vi "Extracted algo.vi"(0 "Image In":T2, 2 "Match Options (Shape Detection 1)":T1={"Rotation"=FALSE, "Scale"=FALSE, "Occlusion"=TRUE, "Range Settings"=[{"Match Constraints"=2, "Min"=0.0, "Max"=50.0}]} {"Range Settings"."Match Constraints" items=["Rotation Angle (degrees)", "Scale Factor (%)", "Occlusion (%)"]}, 3 "Range (Threshold 1)":cluster{"Lower value":sgl, "Upper value":sgl}={"Lower value"=0.0, "Upper value"=195.0}, 7 "error in":errorcluster) -> (20 "Image Out":T2, 21 "Circles (Shape Detection 1)":T3(array[cluster]) {"Position"."Y" format="%.2f"; "Position"."X" format="%.2f"}, 22 "Circles Calibrated (Shape Detection 1)":T3(array[cluster]) {"Position"."Y" format="%.2f"; "Position"."X" format="%.2f"}, 23 "Number of Matches (Shape Detection 1)":i32, 27 "error out":errorcluster)   [LabVIEW 2015]
doc: "Creates, edits, and runs vision algorithms using NI Vision Assistant.\n\nWhen you place this Express VI on the block diagram, NI Vision Assistant launches. Create an algorithm using the Vision Assistant processing functions. After you create an algorithm, you can select the controls and indicators that you want to be able to programmatically set in LabVIEW. Double-click the Vision Assistant Express VI to edit the algorithm."
uses:
  <vilib>/vision/Image Controls.llb/IMAQ Image.ctl
  algo1.vi
  <vilib>/vision/NI_Vision_Development_Module.lvlib
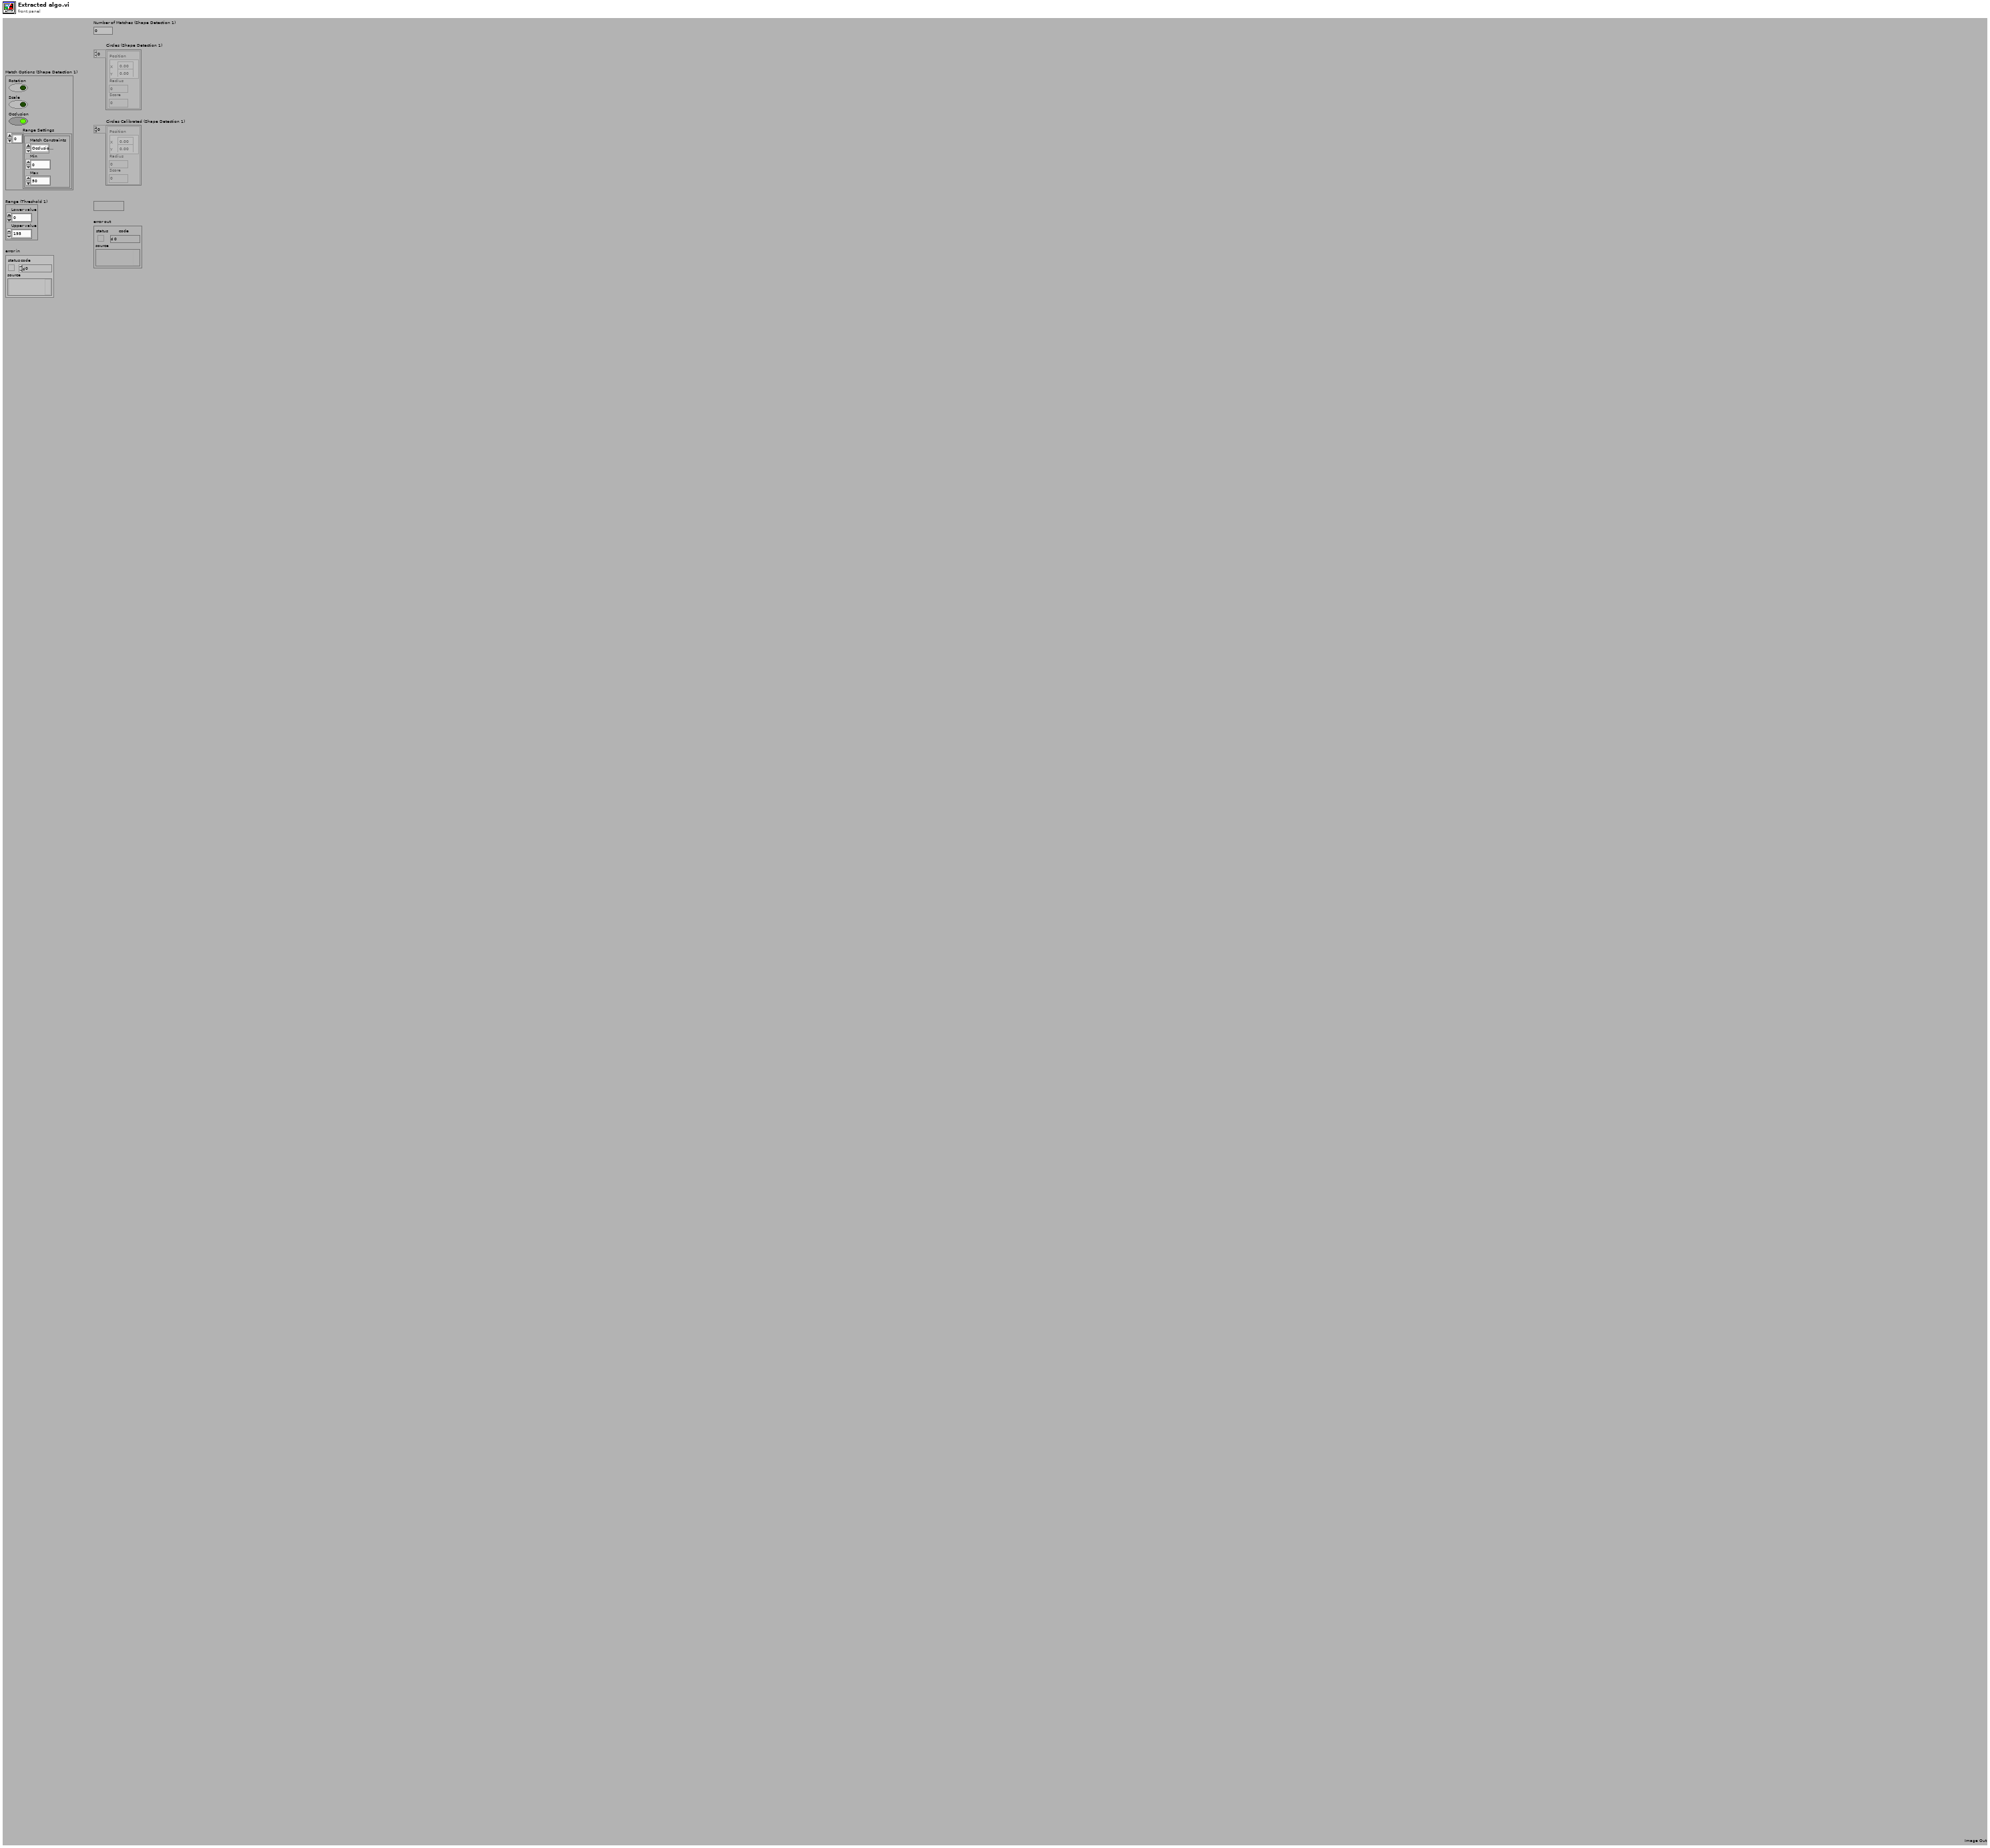
[diagram p1: front panel]
types:
  T1 = cluster{"Rotation":bool, "Scale":bool, "Occlusion":bool, "Range Settings":cluster{"Match Constraints":u32, "Min":dbl, "Max":dbl}[]}
  T2 = typedef "IMAQ Image.ctl" = refnum<image>
  T3 = cluster{"Position":cluster{"X":sgl, "Y":sgl}, "Radius":dbl, "Score":dbl}[]
  T4 = cluster{"Extraction Mode":u32, "Edge Threshold":i32, "Edge Filter Size":u32, "Min Length":i32, "Row Search Step Size":i32, "Col Search Step Size":i32, "Max Endpoint Gap":i32, "Closed":bool, "Subpixel":bool}
  T5 = cluster{"Global Rectangle":i32[], "Contours":cluster{"ID":enum32{"External", "Internal"}, "Type":u32, "Coordinates":i32[]}[]}
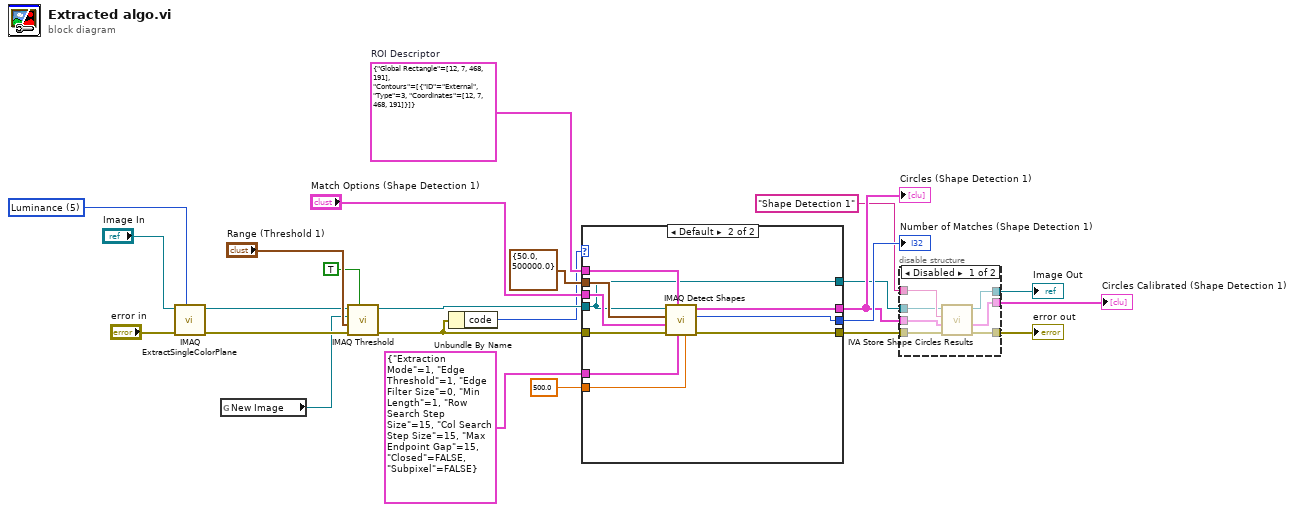
[diagram p0: block diagram]
diagram:
  w13 = T5 {"Global Rectangle"=[12, 7, 468, 191], "Contours"=[{"ID"=enum."External", "Type"=3, "Coordinates"=[12, 7, 468, 191]}]}  # ROI Descriptor
  w24 = 5 items=["Red", "Green", "Blue", "Hue", "Saturation", "Luminance", "Value", "Intensity"] ("Color Plane")
  n1 = call "IMAQ ExtractSingleColorPlane"("Color Plane"=w24, "error in (no error)"="error in", "Image Src"="Image In") -> ("error out"=w22:errorcluster, "Image Dst Out"=w20:T2)  [unwired: 1 in, 6 out]
  n2 = global read "algo1.vi" "New Image"() -> (w1:T2)
  n3 = call "IMAQ Threshold"("Keep/Replace Value (Replace)"=TRUE, "error in (no error)"=w22, "Range"="Range (Threshold 1)", "Image Dst"=w1, "Image Src"=w20) -> ("error out"=w19:errorcluster, "Image Dst Out"=w11:T2)  [unwired: 1 in, 4 out]
  n4 = Unbundle By Name(w19) -> ("code"=w6:i32)
  n5 = case shown="Default" w6 {
    tunnel: w19 -> [_ w35]
    tunnel: [_ w34] -> w18
    tunnel: "Match Options (Shape Detection 1)" -> [_ w33]
    tunnel: T4 {"Extraction Mode"=1, "Edge Threshold"=1, "Edge Filter Size"=0, "Min Length"=1, "Row Search Step Size"=15, "Col Search Step Size"=15, "Max Endpoint Gap"=15, "Closed"=FALSE, "Subpixel"=FALSE} ("Curve Parameters") -> [_ w32]
    tunnel: 500.0 ("Minimum match score") -> [_ w31]
    tunnel: cluster{"Min Radius":dbl, "Max Radius":dbl} {"Min Radius"=50.0, "Max Radius"=500000.0} ("Circle Descriptor") -> [_ w30]
    tunnel: w13 -> [_ w29]
    tunnel: [_ w28] -> w12
    tunnel: w11 -> [w25 w26]
    tunnel: [_ w27] -> w10
    tunnel: [w25 w26] -> w5
    frame -1074396199, -1074396198 {
      # "Discard Coordinate\nSystem Error"
    }
    frame Default {
      n6 = call-poly "IMAQ Detect Shapes"("Minimum match score"=w31, "Curve Parameters"=w32, "ROI Descriptor"=w29, "error in (no error)"=w35, "Match Options"=w33, "Circle Descriptor"=w30, "Image"=w26) -> ("error out"=w27:errorcluster, "Number of Matches Returned"=w34:i32, "Circles"=w28:T3)  [unwired: 2 out]
    }
  }
  "Number of Matches (Shape Detection 1)" <- w18
  "Circles (Shape Detection 1)" <- w12
  n7 = disable-structure shown="Disabled" {
    disable-tunnel: w12 -> [w42 _]
    disable-tunnel: w10 -> [w41 w43]
    disable-tunnel: [w40 w43] -> w9
    disable-tunnel: [w39 _] -> w8
    disable-tunnel: "Shape Detection 1" ("Step Name") -> [w38 _]
    disable-tunnel: w5 -> [w37 w44]
    disable-tunnel: [w36 w44] -> w4
    frame Disabled {
      n8 = call <vilib>:"IVA Store Shape Circles Results.vi"("error in (no error)"=w41, "Circles"=w42, "Step Name"=w38, "Image in"=w37) -> ("error out"=w40:errorcluster, "Circles (Calibrated)"=w39:T3, "Image dup"=w36:T2)  [unwired: 5 out]
    }
    frame Enabled {
    }
  }
  "Circles Calibrated (Shape Detection 1)" <- w8
  "error out" <- w9
  "Image Out" <- w4
